vi "Init.vi"() -> (0 "MQTT_API out":refnum<class "MQTT_API.lvclass">)   [LabVIEW 2019]
uses:
  <vilib>/addons/WireFlow/_WireQueue/MQTT API/MQTT_API.lvclass
  <vilib>/addons/WireFlow/_WireQueue/MQTT API/typedefs/MQTT_ConnectionDetails.ctl
  <vilib>/addons/WireFlow/_WireQueue/MQTT API/typedefs/MQTT_ComSetup.ctl
  <vilib>/addons/WireFlow/_WireQueue/MQTT API/typedefs/MQTT_ComType.ctl
  <vilib>/addons/WireFlow/_WireQueue/MQTT API/typedefs/MQTT_TLS-Conf.ctl
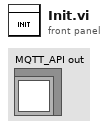
[diagram p1: front panel]
types:
  T1 = typedef "WF_WireQueue-MQTT.lvlib/MQTT_API.lvclass/MQTT_ComSetup.ctl" = cluster{"Communication type":T2, "TLS level (Full TLS)":T3, "TCP_NO-DELAY":bool}
  T2 = typedef "WF_WireQueue-MQTT.lvlib/MQTT_API.lvclass/MQTT_ComType.ctl" = enum16{"TCP/IP", "TCP/IP (TLS)"}
  T3 = typedef "WF_WireQueue-MQTT.lvlib/MQTT_API.lvclass/MQTT_TLS-Conf.ctl" = enum16{"Allow Self-signed crt", "Don't check server name", "Full TLS check"}
  T4 = typedef "WF_WireQueue-MQTT.lvlib/MQTT_API.lvclass/MQTT_ConnectionDetails.ctl" = cluster{"Server address":string, "Server port":u16, "User name":string, "Password":string, "Keep alive time (10 s)":u16, "Reconnect period (20 s)":u16, "Clean session reconnect?":bool}
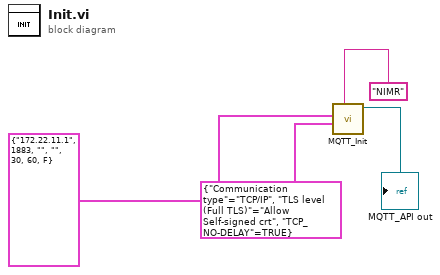
[diagram p0: block diagram]
diagram:
  n1 = call <vilib>:"MQTT_Init.vi"("Client ID"="NIMR", "Communication setup"=T1 {"Communication type"=enum."TCP/IP", "TLS level (Full TLS)"=enum."Allow Self-signed crt", "TCP_NO-DELAY"=TRUE}, "Connection details"=T4 {"Server address"="172.22.11.1", "Server port"=1883, "User name"="", "Password"="", "Keep alive time (10 s)"=30, "Reconnect period (20 s)"=60, "Clean session reconnect?"=FALSE}) -> ("MQTT_API out"=→"MQTT_API out":refnum<class "MQTT_API.lvclass">)  [unwired: 7 in, 1 out]
